vi "string extract.vi"(5 "输入的串":string) -> (0 "输出的串":string, 1 "剩余的串":string, 2 "输出的串非空":bool, 3 "输出数据长度":dbl, 4 "舍弃的串":string)   [LabVIEW 2014]
panel:
  in  "测试用数组(十六进制)":u8[](array[numeric]) format="%#x"
  # "如果要测试功能，建议用十六进制数组替代输入的串。"
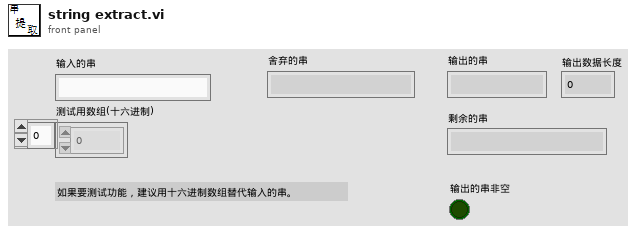
[diagram p1: front panel]
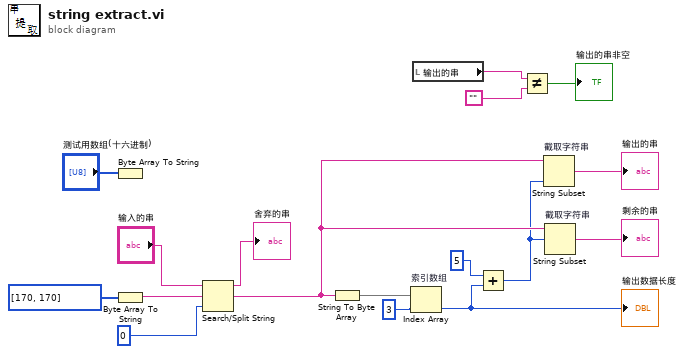
[diagram p0: block diagram]
diagram:
  n1 = Byte Array To String(unsigned byte array="测试用数组(十六进制)") -> ()  [unwired: 1 out]
  n2 = Byte Array To String(unsigned byte array=i32[] [170, 170]) -> (string=w8:string)
  n3 = Search/Split String ("搜索/拆分字符串")(string="输入的串", search string/char (-)=w8, offset (0)=0) -> (substring before match=→"舍弃的串":string, match + rest of string=w10:string)  [unwired: 1 out]
  n4 = String To Byte Array ("字符串至字节数组转换")(string=w10) -> (unsigned byte array=w15:u8[])
  n5 = Index Array "索引数组"(array=w15, index=3) -> (element=w2:u8)
  "输出数据长度" <- w2
  n6 = local read "输出的串"() -> (w7:string)
  n7 = Add(x=5, y=w2) -> (x+y=w1:i32)
  n8 = Not Equal?(x=w7, y="") -> (x != y?=→"输出的串非空":bool)
  n9 = String Subset "截取字符串"(string=w10, length (rest)=w1) -> (substring=→"输出的串":string)  [unwired: 1 in]
  n10 = String Subset "截取字符串"(string=w10, offset (0)=w1) -> (substring=→"剩余的串":string)  [unwired: 1 in]
